vi "Validate Message Refnum.vi"(8 "error in (no error)":errorcluster, 11 "Message in":T1 format="%.0x") -> (0 "error out":errorcluster, 3 "Message out":T1 format="%.0x")   [LabVIEW 2020, in "Instrument Addon Scripting API.lvlib"]
uses:
  Instrument Addon Scripting API.lvlib
  <vilib>/NI VeriStand/Custom Device API/Custom Device Item Ref.ctl
  Addon/Addon Shared/SubVIs/Constants.vi
  Addon/Addon Shared/Instrument Addon Shared.lvlib
  <vilib>/NI VeriStand/Custom Device API/Custom Device API.lvlib
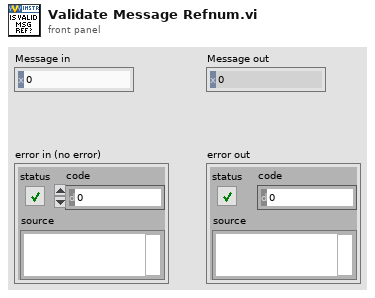
[diagram p1: front panel]
types:
  T1 = typedef "Custom Device API.lvlib/Custom Device Item Ref.ctl" = u64
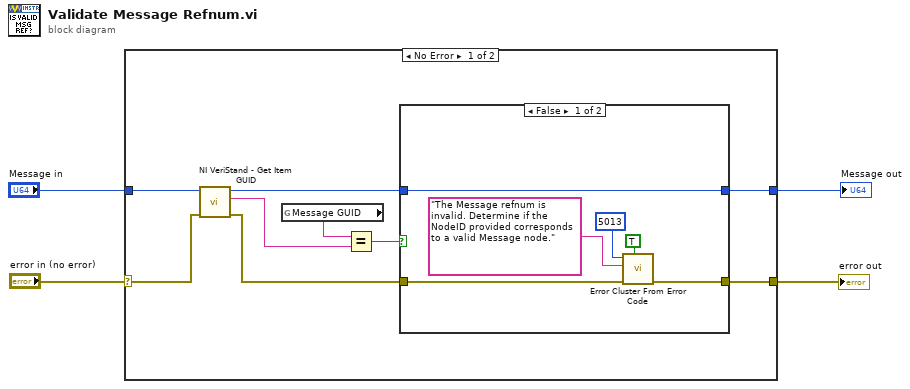
[diagram p0: block diagram]
diagram:
  n1 = case shown="No Error" "error in (no error)" {
    selector: "error in (no error)" -> [w5 w23]
    tunnel: "Message in" -> [w11 w22]
    tunnel: [w7 w22] -> w3
    tunnel: [w6 w23] -> w2
    frame No Error {
      n2 = call <vilib>:"NI VeriStand - Get Item GUID.vi"("error in (no error)"=w5, "Item Ref in"=w11) -> ("error out"=w8:errorcluster, "GUID"=w12:string, "Item Ref out"=w9:T1)  [unwired: 7 in]
      n3 = global read "Constants.vi" "Message GUID"() -> (w13:string)
      n4 = Equal?(x=w13, y=w12) -> (x = y?=w10:bool)
      n5 = case shown="False" w10 {
        tunnel: w9 -> [w18 w21]
        tunnel: w8 -> [w19 w20]
        tunnel: [w18 w21] -> w7
        tunnel: [w17 w20] -> w6
        frame False {
          n6 = call <vilib>:"Error Cluster From Error Code.vi"("show call chain? (False)"=TRUE, "error in (no error)"=w19, "error message (\"\")"="The Message refnum is invalid. Determine if the NodeID provided corresponds to a valid Message node." ("error message (\"\")"), "error code (0)"=5013) -> ("error out"=w17:errorcluster)  [unwired: 5 in]
        }
        frame True {
        }
      }
    }
    frame Error {
    }
  }
  "error out" <- w2
  "Message out" <- w3
